vi "TPNT_GetDeviceData.vi"(8 "error in (no error)":errorcluster, 11 "Object Refnum In":T6) -> (0 "error out":errorcluster, 2 "Object Data Out":T1={"device"="", "devupdate"=0.0, "next_update"=0, "devinterface"="", "TPs"=[], "Alarms"=TRUE, "monitor"=TRUE, "log sep"=""} {"TPs"."Log"."updaterate" format="%.2f"; "TPs"."Samples"."Values" format="%.2f"; "TPs"."Samples"."samples" min=1 step=1; "TPs"."Limits"."Nominal" format="%.2f"; "TPs"."Limits"."Upper" format="%.2f"; "TPs"."Limits"."Lower" format="%.2f"; "TPs"."update_rate" format="%.2f"; "devupdate" format="%.2f"}, 3 "Data Refnum out":T6)   [LabVIEW 2016]
uses:
  TPNT_Refnum.ctl
  TPNT_DeviceTPs.ctl
  TPNT_TP.ctl
  TPNT_Limits.ctl
  TPNT_Samples.ctl
  TPNT_Log.ctl
  TPNT_CoreFunction.ctl
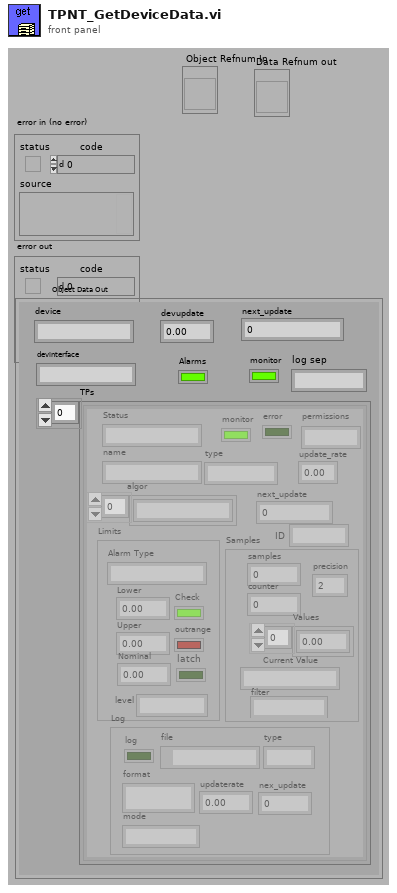
[diagram p1: front panel]
types:
  T1 = typedef "TPNT_DeviceTPs.ctl" = cluster{"device":string, "devupdate":dbl, "next_update":u32, "devinterface":string, "TPs":T2[], "Alarms":bool, "monitor":bool, "log sep":string}
  T2 = typedef "TPNT_TP.ctl" = cluster{"name":string, "type":string, "algor":string[], "update_rate":sgl, "Limits":T3, "Samples":T4, "next_update":u32, "Status":string, "monitor":bool, "error":bool, "Log":T5, "permissions":string, "ID":string}
  T3 = typedef "TPNT_Limits.ctl" = cluster{"Alarm Type":string, "Lower ":dbl, "Upper":dbl, "Nominal":dbl, "outrange":bool, "Check":bool, "latch":bool, "level":string}
  T4 = typedef "TPNT_Samples.ctl" = cluster{"samples":i32, "counter":i32, "Values":dbl[], "Current Value":string, "filter":string, "precision":u8}
  T5 = typedef "TPNT_Log.ctl" = cluster{"log":bool, "file":path, "type":string, "format":string, "updaterate":dbl, "nex_update":u32, "mode":string}
  T6 = typedef "TPNT_Refnum.ctl" = refnum<vi>
  T7 = typedef "TPNT_CoreFunction.ctl" = enum16{"Reset", "Register", "Get Data", "Set Data", "Unregister", "Test", "Get Objects"}
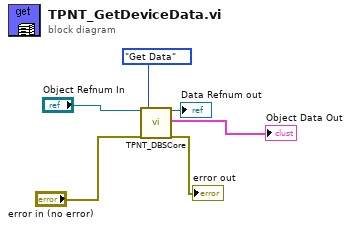
[diagram p0: block diagram]
diagram:
  n1 = call "TPNT_DBSCore.vi"("Object Refnum In"="Object Refnum In", "error in (no error)"="error in (no error)", "Function (Get Data)"=TPNT_CoreFunction."Get Data") -> ("Object Refnum out"=→"Data Refnum out":T6, "Object Data Out"=→"Object Data Out":T1, "error out"=→"error out":errorcluster)  [unwired: 2 in, 12 out]
